vi "Append PDF files to PDF Report  GetImportedPage.vi"(0 "PDF Report":refnum<class "PDF Report Class.lvclass">, 7 "PDF Files  to concatenate":T1={"Path"=path "", "Pages"="all", "Password"=""}, 11 "error in (no error)":errorcluster) -> (4 "PDF Report duplicate":refnum<class "PDF Report Class.lvclass">, 15 "error out":errorcluster)   [LabVIEW 2019, in "Exaprom PDF.lvlib"]
doc: "We use PDF Writer to import a page: All interactive features (annotations, bookmarks, fields, and so forth) of the imported page are lost in the process. The size of the imported page could be reduced to fit in the page of the PDF Report.\n\nVersion 1.0\nDeveloped by Jean-Marc Simard\nCopyright © 2012, Exaprom Inc.\nAll rights reserved.\nLicense: BSD\n\nWith iTextSharp Library\n(http://itextsharp.sourceforge.net)"
uses:
  LV Class/PDF Report Class/PDF Report Class.lvclass
  Controls/Concatenate Controls/PDF file to concatenate.ctl
  Controls/General Controls/Create, open or close.ctl
  C:/work/niobrara_lv/labview pdf writer fixing/DLL/itextsharp.dll
  DLL/itextsharp.dll
  Exaprom PDF.lvlib
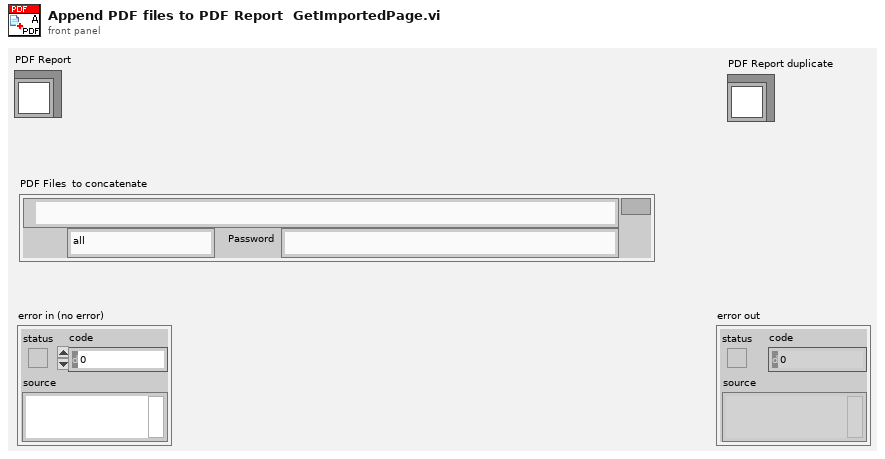
[diagram p1: front panel]
types:
  T1 = typedef "Exaprom PDF.lvlib/PDF file to concatenate.ctl" = cluster{"Path":path, "Pages":string, "Password":string}
  T2 = typedef "Exaprom PDF.lvlib/Create, open or close.ctl" = enum16{"Create", "Open", "Close"}
  T3 = typedef "Exaprom PDF.lvlib/Page dimensions.ctl" = cluster{"Start at page":i32, "Page Size":T4, "Orientation":T5, "widht":sgl, "height":sgl, "Margin left":sgl, "Margin right":sgl, "Margin top":sgl, "Margin bottom":sgl, "X0":sgl, "X1":sgl, "Y0":sgl, "Y1":sgl}
  T4 = typedef "Exaprom PDF.lvlib/Page size.ctl" = i32
  T5 = typedef "Exaprom PDF.lvlib/Page Orientation.ctl" = enum16{"Portrait", "Landscape"}
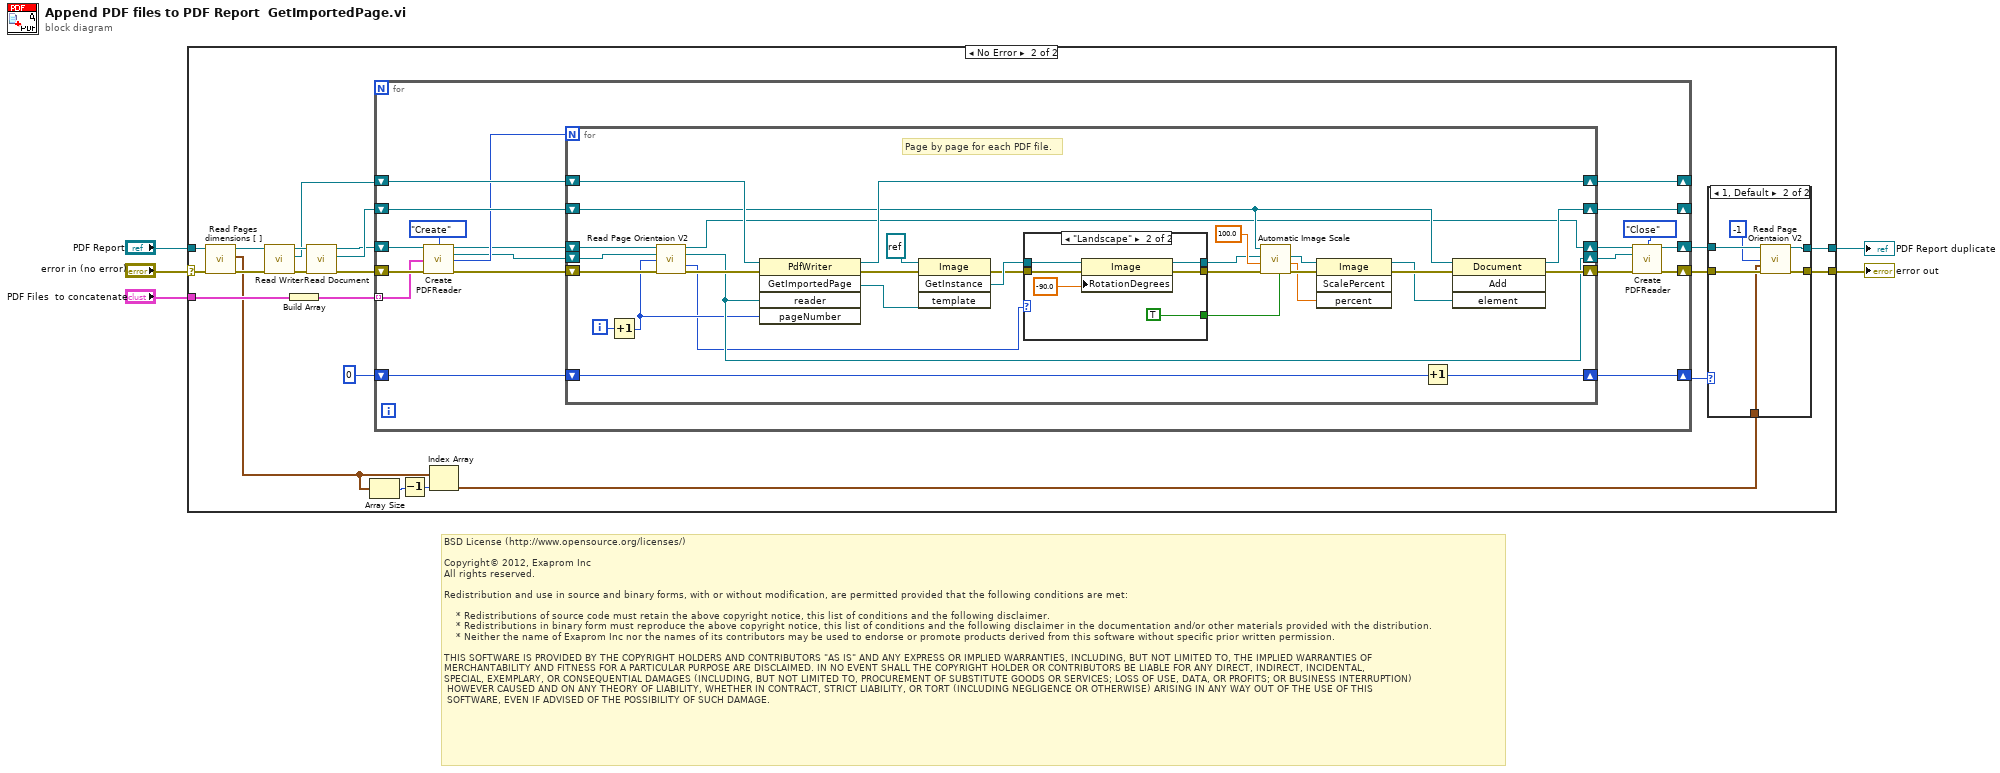
[diagram p0: block diagram]
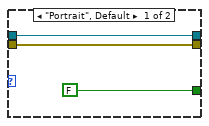
[diagram p4: hidden frame]
diagram:
  # "BSD License (http://www.opensource.org/licenses/)\n\nCopyright© 2012, Exaprom Inc\nAll rights reserved.\n\nRedistribution and use in source and binary forms, with or without modification, are permitted provided that the following conditions are met:\n\n    * Redistributions of source code must retain the above copyright notice, this list of conditions and the following disclaimer.\n    * Redistributions in binary form must reproduce the above copyright notice, this list of conditions and the following disclaimer in the documentation and/or other materials provided with the distribution.\n    * Neither the name of Exaprom Inc nor the names of its contributors may be used to endorse or promote products derived from this software without specific prior written permission.\n\nTHIS SOFTWARE IS PROVIDED BY THE COPYRIGHT HOLDERS AND CONTRIBUTORS \"AS IS\" AND ANY EXPRESS OR IMPLIED WARRANTIES, INCLUDING, BUT NOT LIMITED TO, THE IMPLIED WARRANTIES OF \nMERCHANTABILITY AND FITNESS FOR A PARTICULAR PURPOSE ARE DISCLAIMED. IN NO EVENT SHALL THE COPYRIGHT HOLDER OR CONTRIBUTORS BE LIABLE FOR ANY DIRECT, INDIRECT, INCIDENTAL,\nSPECIAL, EXEMPLARY, OR CONSEQUENTIAL DAMAGES (INCLUDING, BUT NOT LIMITED TO, PROCUREMENT OF SUBSTITUTE GOODS OR SERVICES; LOSS OF USE, DATA, OR PROFITS; OR BUSINESS INTERRUPTION)\n HOWEVER CAUSED AND ON ANY THEORY OF LIABILITY, WHETHER IN CONTRACT, STRICT LIABILITY, OR TORT (INCLUDING NEGLIGENCE OR OTHERWISE) ARISING IN ANY WAY OUT OF THE USE OF THIS\n SOFTWARE, EVEN IF ADVISED OF THE POSSIBILITY OF SUCH DAMAGE."
  n1 = case shown="No Error" "error in (no error)" {
    selector: "error in (no error)" -> [w7 w20]
    tunnel: [w7 w17] -> w5
    tunnel: "PDF Files  to concatenate" -> [_ w28]
    tunnel: "PDF Report" -> [w6 w21]
    tunnel: [w6 w16] -> w2
    frame Error {
    }
    frame No Error {
      n2 = call-dynamic "Read Pages dimensions [ ].vi"("PDF Report Class in"=w21) -> ("Pages dimensions [ ]"=w11:T3[], "PDF Report Class out"=w14:refnum<class "PDF Report Class.lvclass">)  [unwired: 7 in, 2 out]
      n3 = call-dynamic "Read Writer.vi"("error in (no error)"=w20, "PDF Report Class in"=w14) -> ("error out"=w25:errorcluster, "Writer"=w23:refnum<k24>, "PDF Report Class out"=w24:refnum<class "PDF Report Class.lvclass">)  [unwired: 7 in]
      n4 = Build Array(w28) -> (w8:T1[])
      n5 = call-dynamic "Read Document.vi"("error in (no error)"=w25, "PDF Report Class in"=w24) -> ("error out"=w26:errorcluster, "Document"=w27:refnum<k24>, "PDF Report Class out"=w22:refnum<class "PDF Report Class.lvclass">)  [unwired: 7 in]
      n6 = Array Size(array=w11) -> (size(s)=w13:i32)
      n7 = for {
        shift-right: [w39] -> _
        shift-left: w27 -> [w53]
        shift-right: [w40] -> w18
        shift-left: w26 -> [w52]
        shift-right: [w54] -> _
        shift-left: w23 -> [w56]
        tunnel: w8 -> [w50] mode=indexing
        shift-right: [w41] -> w15
        shift-left: w22 -> [w46]
        shift-right: [w37] -> w9
        shift-left: 0 -> [w38]
        n8 = call "Create PDFReader.vi"("PDF Report IN"=w46, "Action"=Create,_open_or_close."Create", "File and pages"=w50, "error in (no error)"=w52) -> ("PDF Report duplicate"=w45:refnum<class "PDF Report Class.lvclass">, "PdfReader OUT"=w48:refnum<k24>, "NumberOfPages"=w49:i32, "error out"=w51:errorcluster)  [unwired: 8 in]
        n9 = for {
          N: w49 -> [_]
          shift-right: [w77] -> w39
          shift-left: w53 -> [w75]
          shift-right: [w68] -> w44
          shift-left: w48 -> [w69]
          shift-right: [w78] -> w55
          shift-left: w51 -> [w71]
          shift-right: [w81] -> w54
          shift-left: w56 -> [w85]
          shift-right: [w66] -> w42
          shift-left: w45 -> [w67]
          shift-right: [w65] -> w37
          shift-left: w38 -> [w64]
          i -> [w86]
          # "Page by page for each PDF file."
          n10 = Increment(x=w86) -> (x+1=w63:i32)
          n11 = call "Read Page Orientaion V2.vi"("PDF Report IN"=w67, "PdfReader ref"=w69, "PdfReader page number"=w63, "error in (no error)"=w71) -> ("PDF Report OUT"=w66:refnum<class "PDF Report Class.lvclass">, "PdfReader ref duplicate"=w68:refnum<k24>, "Orientation"=w58:T5, "error out"=w70:errorcluster)  [unwired: 8 in]
          n12 = invoke class="PdfWriter" method="GetImportedPage"(reference=w85, error in=w70, "reader"=w68, "pageNumber"=w63) -> (reference out=w81:refnum<k24>, error out=w84:errorcluster, "GetImportedPage"=w83:refnum<k24>)  [unwired: 1 in, 2 out]
          n13 = invoke class="Image" method="GetInstance"(reference=refnum<k24> refnum ("image"), error in=w84, "template"=w83) -> (error out=w61:errorcluster, "GetInstance"=w62:refnum<k24>)  [unwired: 1 in, 2 out]
          n14 = case shown="\"Landscape\"" w58 {
            tunnel: w62 -> [w88 w95]
            tunnel: w61 -> [w89 w94]
            tunnel: [w89 w93] -> w60
            tunnel: [w88 w91] -> w59
            tunnel: [FALSE TRUE] -> w57
            frame "Portrait", Default {
            }
            frame "Landscape" {
              n15 = property class="Image"(reference=w95, error in=w94, "RotationDegrees"=sgl -90.0) -> (reference out=w91:refnum<k24>, error out=w93:errorcluster)
            }
          }
          n16 = call "Automatic Image Scale.vi"("Rotate?"=w57, "error in (no error)"=w60, "Scale percent IN"=sgl 100.0, "GetInstanceImage IN"=w59, "Document"=w75) -> ("error out"=w76:errorcluster, "Scale percent OUT"=w74:sgl, "GetInstanceImage OUT"=w72:refnum<k24>)  [unwired: 2 in, 2 out]
          n17 = invoke class="Image" method="ScalePercent"(reference=w72, error in=w76, "percent"=w74) -> (reference out=w79:refnum<k24>, error out=w80:errorcluster)  [unwired: 1 in, 2 out]
          n18 = Increment(x=w64) -> (x+1=w65:i32)
          n19 = invoke class="Document" method="Add"(reference=w75, error in=w80, "element"=w79) -> (reference out=w77:refnum<k24>, error out=w78:errorcluster)  [unwired: 1 in, 2 out]
        }
        n20 = call "Create PDFReader.vi"("PDF Report IN"=w42, "Action"=Create,_open_or_close."Close", "PdfReader IN"=w44, "error in (no error)"=w55) -> ("PDF Report duplicate"=w41:refnum<class "PDF Report Class.lvclass">, "error out"=w40:errorcluster)  [unwired: 8 in, 2 out]
      }
      n21 = Decrement(x=w13) -> (x-1=w12:i32)
      n22 = Index Array(array=w11, index=w12) -> (element=w10:T3)
      n23 = case shown="1, Default" w9 {
        tunnel: w18 -> [w29 w36]
        tunnel: [w29 w35] -> w17
        tunnel: [w30 w34] -> w16
        tunnel: w15 -> [w30 w33]
        tunnel: w10 -> [_ w31]
        frame 0 {
        }
        frame 1, Default {
          n24 = call "Read Page Orientaion V2.vi"("PDF Report IN"=w33, "PdfReader page number"=-1, "Page (points)"=w31, "error in (no error)"=w36) -> ("PDF Report OUT"=w34:refnum<class "PDF Report Class.lvclass">, "error out"=w35:errorcluster)  [unwired: 8 in, 2 out]
        }
      }
    }
  }
  "error out" <- w5
  "PDF Report duplicate" <- w2
